vi "Practice programming code.vi"() -> ()   [LabVIEW 2013]
panel:
  out "X":i32
  out "Y":i32
  in  "Enum":enum16{"UP", "DOWN", "LEFT", "RIGHT"}(ring)
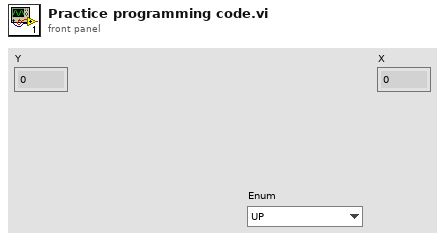
[diagram p1: front panel]
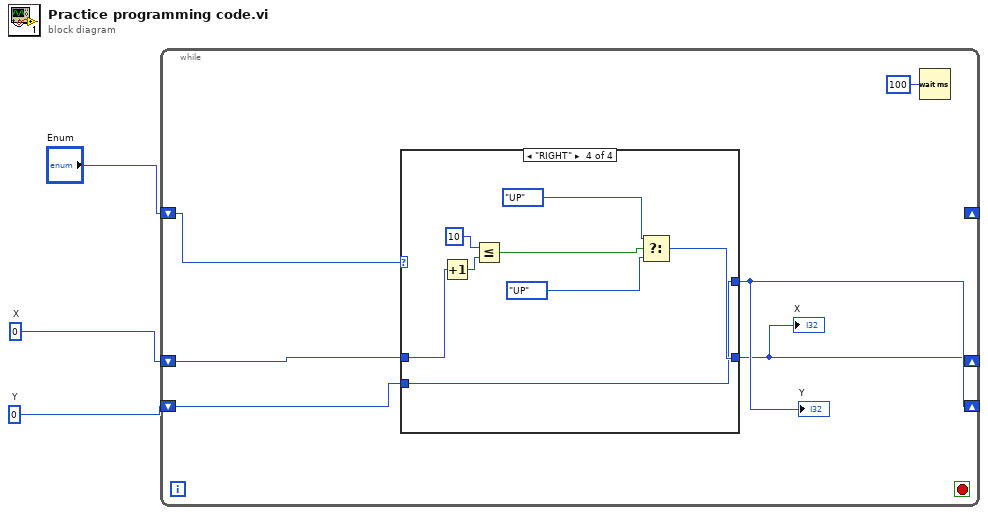
[diagram p0: block diagram]
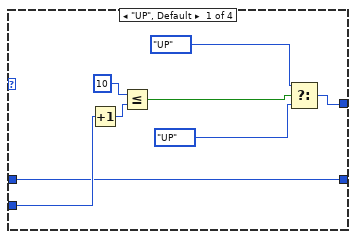
[diagram p2: hidden frame]
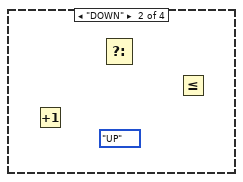
[diagram p3: hidden frame]
diagram:
  w2 = 0  # Y
  w1 = 0  # X
  n1 = while {
    shift-right: _ -> [_]
    shift-left: "Enum" -> [w9]
    shift-right: [w4] -> _
    shift-left: w1 -> [w7]
    shift-right: [w5] -> _
    shift-left: w2 -> [w8]
    stop <- _ stop-if-true
    n2 = case shown="\"RIGHT\"" w9 {
      tunnel: w8 -> [w17 _ _ w18]
      tunnel: w7 -> [w10 _ _ w20]
      tunnel: [w11 _ _ w18] -> w5
      tunnel: [w10 _ _ w19] -> w4
      frame "UP", Default {
        n3 = Increment(x=w17) -> (x+1=w16:i32)
        n4 = Less Or Equal?(x=10, y=w16) -> (x <= y?=w14:bool)
        n5 = Select(t=enum16{"UP", "DOWN", "LEFT", "RIGHT"}."UP" ("Enum 2"), s=w14, f=enum16{"UP", "DOWN", "LEFT", "RIGHT"}."UP" ("Enum 2")) -> (s? t:f=w11:enum16{"UP", "DOWN", "LEFT", "RIGHT"})
      }
      frame "DOWN" {
        (unwired) enum16{"UP", "DOWN", "LEFT", "RIGHT"}."UP" ("Enum 2")
        n6 = Increment() -> ()  [unwired: 1 in, 1 out]
        n7 = Select() -> ()  [unwired: 3 in, 1 out]
        n8 = Less Or Equal?() -> ()  [unwired: 2 in, 1 out]
      }
      frame "LEFT" {
      }
      frame "RIGHT" {
        n9 = Increment(x=w20) -> (x+1=w25:i32)
        n10 = Less Or Equal?(x=10, y=w25) -> (x <= y?=w23:bool)
        n11 = Select(t=enum16{"UP", "DOWN", "LEFT", "RIGHT"}."UP" ("Enum 2"), s=w23, f=enum16{"UP", "DOWN", "LEFT", "RIGHT"}."UP" ("Enum 2")) -> (s? t:f=w19:enum16{"UP", "DOWN", "LEFT", "RIGHT"})
      }
    }
    "Y" <- w5
    "X" <- w4
    n12 = Wait (ms)(milliseconds to wait=u32 100) -> ()  [unwired: 1 out]
  }
